vi "Initialize_Images_Array_Random_Names-2.vi"(2 "error IN":errorcluster, 3 "# Pics":i32, 4 "Image Type":T1 items=["Grayscale (U8)", "Grayscale (I16)", "Grayscale (SGL)", "Complex (CSG)", "RGB (U32)", "HSL (U32)", "RGB (U64)", "Grayscale (U16)"], 5 "Unique ID":string) -> (0 "error OUT":errorcluster, 1 "Images Array":T2[](array[typedef]))   [LabVIEW 2013]
uses:
  <vilib>/vision/Image Controls.llb/IMAQ Image.ctl
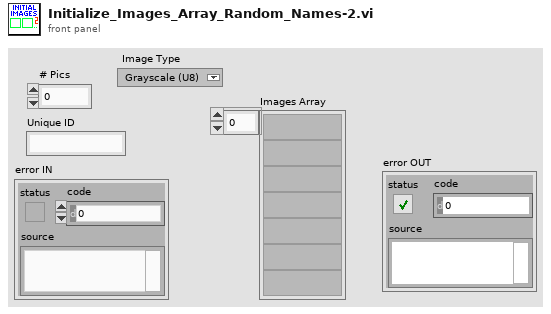
[diagram p1: front panel]
types:
  T1 = typedef "Image Type" = u32
  T2 = typedef "IMAQ Image.ctl" = refnum<image>
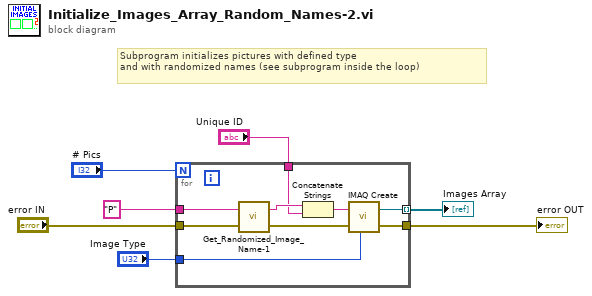
[diagram p0: block diagram]
diagram:
  # "Subprogram initializes pictures with defined type \nand with randomized names (see subprogram inside the loop)"
  n1 = for {
    N: "# Pics" -> [_]
    tunnel: "error IN" -> [w14]
    tunnel: [w16] -> w5 mode=indexing
    tunnel: "Image Type" -> [w15]
    tunnel: "P" ("Main Name") -> [w13]
    tunnel: "Unique ID" -> [w9]
    tunnel: [w8] -> w1
    n2 = call "Get_Randomized_Image_Name-1.vi"("error IN"=w14, "Main Name"=w13) -> ("error OUT"=w12:errorcluster, "Randomized name"=w10:string)
    n3 = Concatenate Strings(w10, w9) -> (w11:string)
    n4 = call "IMAQ Create"("Image Name"=w11, "Image Type"=w15, "error in (no error)"=w12) -> ("New Image"=w16:T2, "error out"=w8:errorcluster)  [unwired: 2 in]
  }
  "Images Array" <- w5
  "error OUT" <- w1
